vi "Create Temp U32.vi"(7 "W[i]":u32, 8 "K":u32, 9 "E":u32, 10 "F":u32, 11 "A":u32) -> (2 "A Out":u32 format="%b", 3 "Temp Out":u32 format="%b")   [LabVIEW 2014]
panel:
  out "x << y":fxp<+,39,39> format="%b"
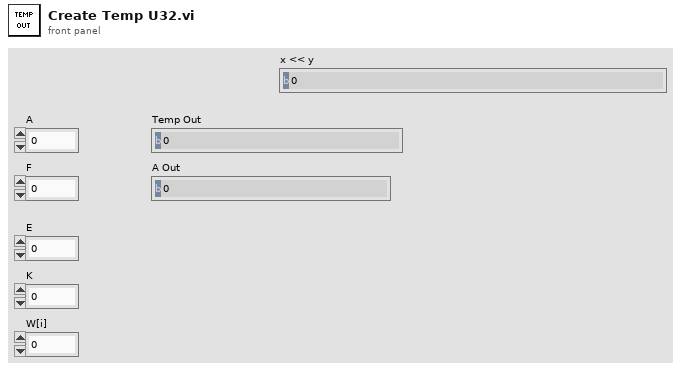
[diagram p1: front panel]
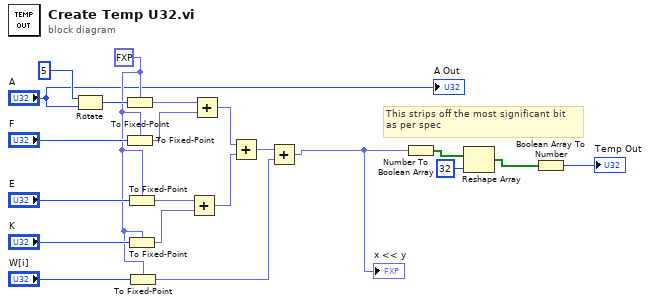
[diagram p0: block diagram]
diagram:
  w8 = fxp<+,33,33> 0.0 ("fixed-point type")
  # "This strips off the most significant bit\nas per spec"
  n1 = Rotate(1:"A", 2:u32 5 ("x")) -> (0:w21:u32)
  n2 = To Fixed-Point(fixed-point type=w8, number=w21) -> (fixed-point=w16:fxp<+,33,33>)
  n3 = To Fixed-Point(fixed-point type=w8, number="F") -> (fixed-point=w15:fxp<+,33,33>)
  n4 = To Fixed-Point(fixed-point type=w8, number="E") -> (fixed-point=w14:fxp<+,33,33>)
  n5 = To Fixed-Point(fixed-point type=w8, number="K") -> (fixed-point=w13:fxp<+,33,33>)
  n6 = To Fixed-Point(fixed-point type=w8, number="W[i]") -> (fixed-point=w9:fxp<+,33,33>)
  n7 = Add(x=w14, y=w13) -> (x+y=w11:fxp<+,34,34>)
  n8 = Add(x=w16, y=w15) -> (x+y=w12:fxp<+,34,34>)
  n9 = Add(x=w12, y=w11) -> (x+y=w10:fxp<+,35,35>)
  n10 = Add(x=w10, y=w9) -> (x+y=w1:fxp<+,36,36>)
  "x << y" <- w1
  n11 = Number To Boolean Array(number=w1) -> (Boolean array=w5:bool[])
  n12 = Reshape Array(w5, 32 ("dimension size")) -> (w3:bool[])
  n13 = Boolean Array To Number(Boolean array=w3) -> (number=→"Temp Out":u32)
  "A Out" <- "A"
